vi "ParseJoystickValues.vi"(9 "JoyRef":T1, 10 "Button Names":T4, 11 "Axis Names":T3) -> (2 "Named Button Values":T4, 3 "Named Axis Values":T3)   [LabVIEW 2014]
uses:
  OpAxis.ctl
  OpButtons.ctl
  <vilib>/Rock Robotics/WPI/Joystick/WPI_JoystickDevRef.ctl
  <vilib>/Rock Robotics/WPI/Joystick/WPI_JoystickDeviceEnum.ctl
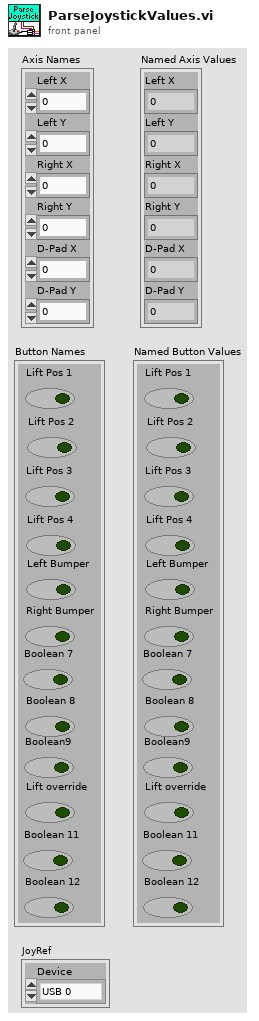
[diagram p1: front panel]
types:
  T1 = typedef "WPI_JoystickDevRef.ctl" = cluster{"Device":T2}
  T2 = typedef "WPI_JoystickDeviceEnum.ctl" = enum16{"USB 0", "USB 1", "USB 2", "USB 3", "USB 4", "USB 5"}
  T3 = typedef "OpAxis.ctl" = cluster{"Left X":dbl, "Left Y":dbl, "Right X":dbl, "Right Y":dbl, "D-Pad X":dbl, "D-Pad Y":dbl}
  T4 = typedef "OpButtons.ctl" = cluster{"Lift Pos 1":bool, "Lift Pos 2":bool, "Lift Pos 3":bool, "Lift Pos 4":bool, "Left Bumper":bool, "Right Bumper":bool, "Boolean 7":bool, "Boolean 8":bool, "Boolean9":bool, "Lift override":bool, "Boolean 11":bool, "Boolean 12":bool}
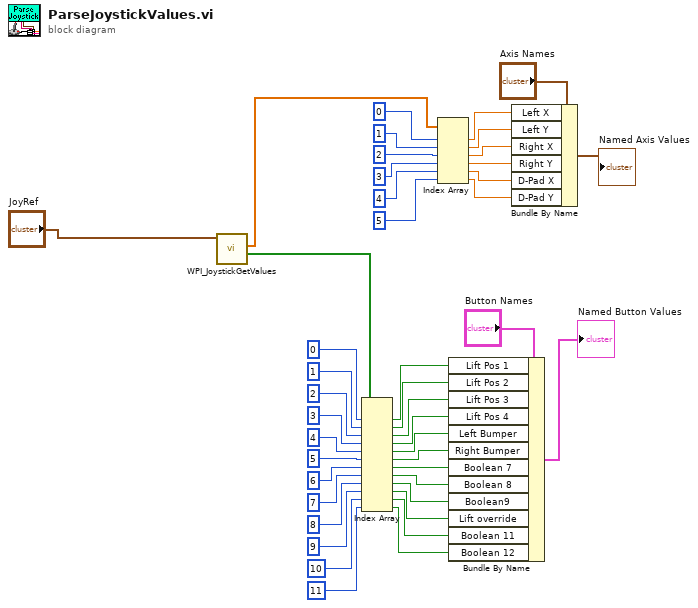
[diagram p0: block diagram]
diagram:
  n1 = call <vilib>:"WPI_JoystickGetValues.vi"("JoystickDevRef"="JoyRef") -> ("Buttons"=w40:bool[], "Axes"=w13:dbl[])  [unwired: 6 in, 3 out]
  n2 = Index Array(array=w40, index #1=0 ("index"), index #2=1 ("index"), index #3=2 ("index"), index #4=3 ("index"), index #5=4 ("index"), index #6=5 ("index"), index #7=6 ("index"), index #8=7 ("index"), index #9=8 ("index"), index #10=9 ("index"), index #11=10 ("index"), index #12=11 ("index")) -> (element #1=w28:bool, element #2=w29:bool, element #3=w30:bool, element #4=w31:bool, element #5=w32:bool, element #6=w33:bool, element #7=w34:bool, element #8=w35:bool, element #9=w36:bool, element #10=w37:bool, element #11=w38:bool, element #12=w39:bool)
  n3 = Index Array(array=w13, index #1=0 ("index"), index #2=1 ("index"), index #3=2 ("index"), index #4=3 ("index"), index #5=4 ("index"), index #6=5 ("index")) -> (element #1=w7:dbl, element #2=w8:dbl, element #3=w9:dbl, element #4=w10:dbl, element #5=w11:dbl, element #6=w12:dbl)
  n4 = Bundle By Name(cluster="Button Names", "Lift Pos 1"=w28, "Lift Pos 2"=w29, "Lift Pos 3"=w30, "Lift Pos 4"=w31, "Left Bumper"=w32, "Right Bumper"=w33, "Boolean 7"=w34, "Boolean 8"=w35, "Boolean9"=w36, "Lift override"=w37, "Boolean 11"=w38, "Boolean 12"=w39) -> (→"Named Button Values":T4)
  n5 = Bundle By Name(cluster="Axis Names", "Left X"=w7, "Left Y"=w8, "Right X"=w9, "Right Y"=w10, "D-Pad X"=w11, "D-Pad Y"=w12) -> (→"Named Axis Values":T3)
